vi "Untitled 2.vi"() -> ()   [LabVIEW 2023]
panel:
  out "Settings":T1
  out "JSON string":string
  in  "Heater":cluster{"P":dbl, "I":dbl} caption="Нагреватель" {"I" format="%#_f"; "P" format="%#_f"}
  in  "PLC2":cluster{"port":u16, "address":string}
  in  "PLC1":cluster{"port":u16, "address":string}
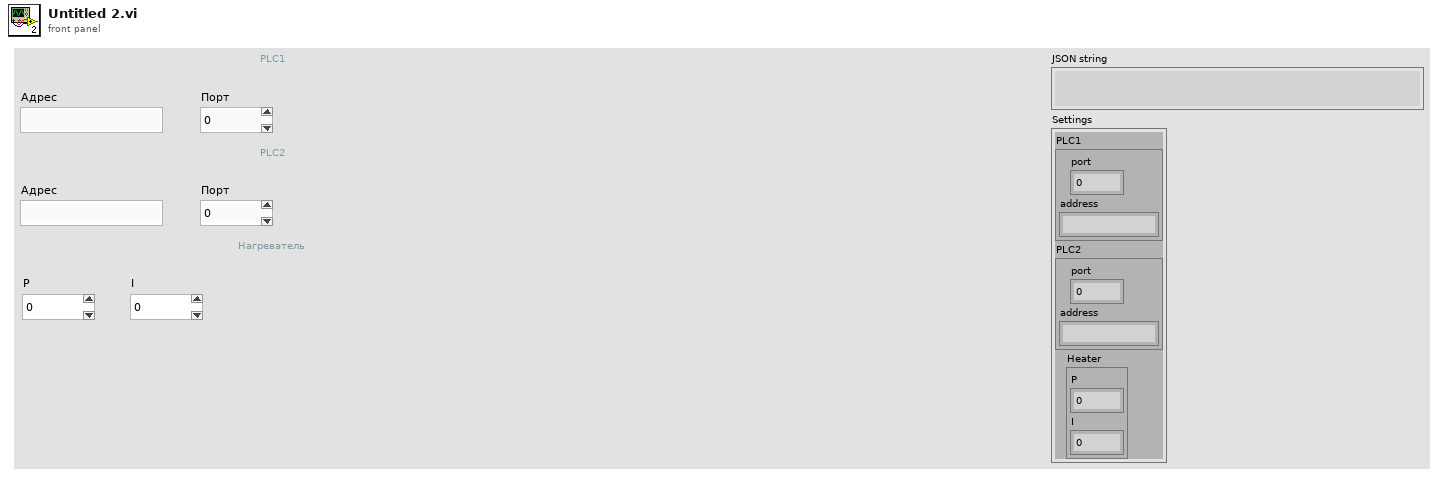
[diagram p1: front panel]
types:
  T1 = cluster{"PLC1":cluster{"port":u16, "address":string}, "PLC2":cluster{"port":u16, "address":string}, "Heater":cluster{"P":dbl, "I":dbl}}
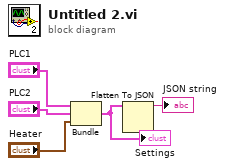
[diagram p0: block diagram]
diagram:
  n1 = Bundle("PLC1"="PLC1", "PLC2"="PLC2", "Heater"="Heater") -> (w2:T1)  [unwired: 1 in]
  "Settings" <- w2
  n2 = Flatten To JSON(anything=w2) -> (JSON string=→"JSON string":string)  [unwired: 2 in, 1 out]
